vi "ma_Tone estimation (FFT input) (CDB).vi"(10 "spectral info":T1 {"window" items=["Rectangle"=0, "Hanning"=1, "Hamming"=2, "Blackman-Harris"=3, "Exact Blackman"=4, "Blackman"=5, "Flat Top"=6, "4 Term B-Harris "=7, "7 Term B-Harris"=8, "Low Sidelobe"=9, "Blackman Nuttall"=11, "Triangle"=30, "Bartlett-Hanning"=31, "Bohman"=32, "Parzen"=33, "Welch"=34, "Kaiser"=60, "Dolph-Chebyshev"=61, "Gaussian"=62]}, 11 "three fingers":T3={"f0"=0.0, "df"=1.0, "spectrum"=[]} {"spectrum" format="%.2f"; "df" format="%.2f"; "f0" format="%.2f"}) -> (3 "single tone info.":T2 {"phase [degree]" format="%.2f"; "amplitude" format="%.2f"; "frequency" format="%.5f"})   [LabVIEW 2020, in "NI_MAPro.lvlib"]
uses:
  NI_MAPro.lvlib
  ma_sml_Spectrum Cluster (complex).ctl
  ma_sml_Spectral Info.ctl
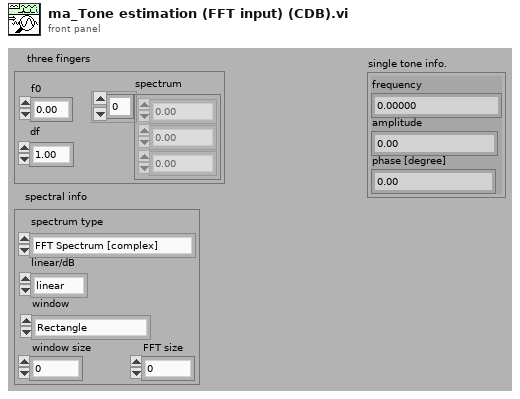
[diagram p1: front panel]
types:
  T1 = typedef "NI_MAPro.lvlib/ma_sml_Spectral Info.ctl" = cluster{"spectrum type":enum16{"FFT Spectrum [complex]", "Amplitude [Magnitude]", "Power [Magnitude^2]", "Cross Spectrum [complex]", "Frequency Response [Complex]"}, "linear/dB":enum16{"linear", "dB"}, "window":u16, "window size":i32, "FFT size":i32}
  T2 = cluster{"frequency":dbl, "amplitude":dbl, "phase [degree]":dbl}
  T3 = typedef "NI_MAPro.lvlib/ma_sml_Spectrum Cluster (complex).ctl" = cluster{"f0":dbl, "df":dbl, "spectrum":cdb[]}
  T4 = cluster{"initial guess frequency":dbl, "Amplitude":dbl, "phase [degree]":dbl}
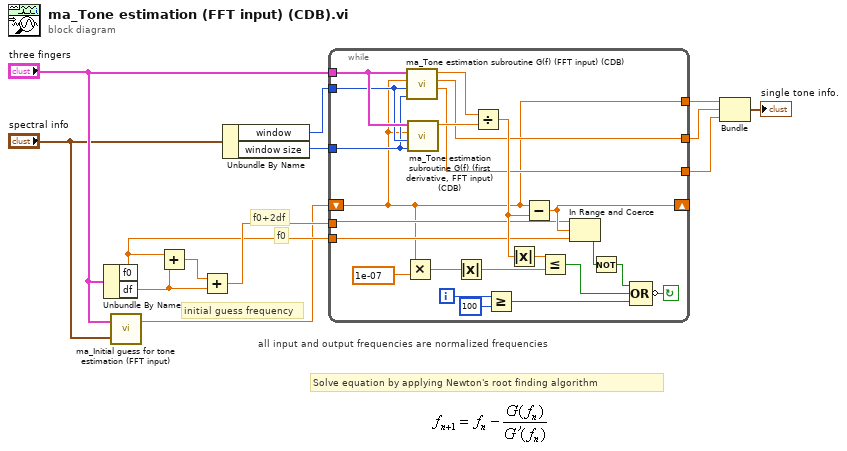
[diagram p0: block diagram]
diagram:
  # "initial guess frequency"
  # "f0"
  # "f0+2df"
  # "Solve equation by applying Newton's root finding algorithm"
  # "all input and output frequencies are normalized frequencies"
  n1 = Unbundle By Name("three fingers") -> ("f0"=w5:dbl, "df"=w7:dbl)
  n2 = call "ma_Initial guess for tone estimation (FFT input).vi"("spectral info"="spectral info", "three fingers"="three fingers") -> ("initial guess frequency"=w1:dbl)  [unwired: 1 out]
  n3 = Add(x=w5, y=w7) -> (x+y=w4:dbl)
  n4 = Add(x=w4, y=w7) -> (x+y=w6:dbl)
  n5 = Unbundle By Name("spectral info") -> ("window"=w9:u16, "window size"=w10:i32)
  n6 = while {
    tunnel: "three fingers" -> [w21]
    tunnel: w5 -> [w22]
    tunnel: w10 -> [w19]
    tunnel: w9 -> [w20]
    tunnel: w6 -> [w23]
    tunnel: [w29] -> w12
    tunnel: [w30] -> w11
    tunnel: [w17] -> w8
    shift-left: w1 -> [w17]
    shift-right: [w26] -> _
    i -> [w31]
    stop <- w33 continue-if-true
    n7 = Multiply(x=w17, y=1e-07) -> (x*y=w16:dbl)
    n8 = call "ma_Tone estimation subroutine G(f) (FFT input) (CDB).vi"("N (window length)"=w19, "window"=w20, "frequency"=w17, "three fingers"=w21) -> ("phase [degree]"=w29:dbl, "Amplitude"=w30:dbl, "G(f)"=w27:dbl)  [unwired: 5 out]
    n9 = call "ma_Tone estimation subroutine G(f) (first derivative, FFT input) (CDB).vi"("N (window length)"=w19, "window"=w20, "frequency"=w17, "three fingers"=w21) -> ("G'(f)"=w36:dbl)  [unwired: 7 out]
    n10 = Absolute Value(x=w16) -> (abs(x)=w14:dbl)
    n11 = Divide(x=w27, y=w36) -> (x/y=w32:dbl)
    n12 = Greater Or Equal?(x=w31, y=100) -> (x >= y?=w34:bool)
    n13 = Absolute Value(x=w32) -> (abs(x)=w35:dbl)
    n14 = Subtract(x=w17, y=w32) -> (x-y=w26:dbl)
    n15 = Less Or Equal?(x=w35, y=w14) -> (x <= y?=w28:bool)
    n16 = In Range and Coerce(upper limit=w23, x=w26, lower limit=w22) -> (In Range?=w24:bool)  [unwired: 1 out]
    n17 = Not(x=w24) -> (.not. x?=w25:bool)
    n18 = Compound Arithmetic op=OR(w25, w28, w34) -> (invert w33:bool)
  }
  n19 = Bundle("initial guess frequency"=w8, "Amplitude"=w11, "phase [degree]"=w12) -> (→"single tone info.":T4)  [unwired: 1 out]
